vi "Lab_2.vi"() -> ()   [LabVIEW 2021]
panel:
  out "C":dbl[][](array[numeric])
  out "B":dbl[][](array[numeric])
  out "A":dbl[][](array[numeric])
  out "Mo":dbl[][](array[numeric])
  out "Con":dbl[][](array[numeric])
  out "MC":dbl[][](array[numeric])
  in  "b4":dbl
  in  "b3":dbl
  in  "b2":dbl
  in  "b1":dbl
  in  "a4":dbl
  in  "a3":dbl
  in  "a2":dbl
  in  "a1":dbl
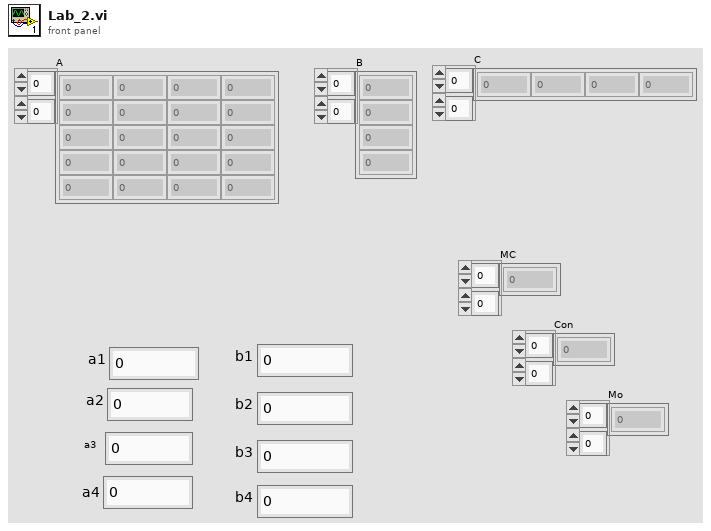
[diagram p1: front panel]
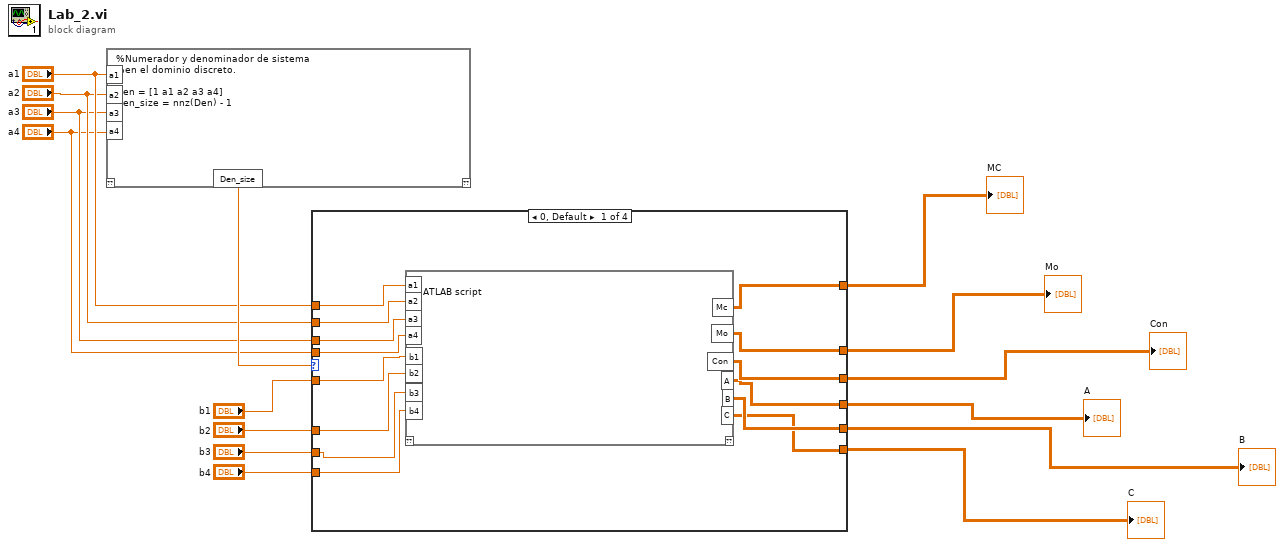
[diagram p0: block diagram]
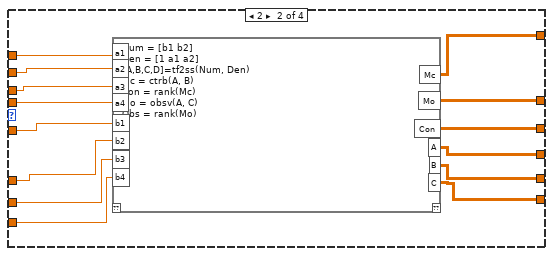
[diagram p2: hidden frame]
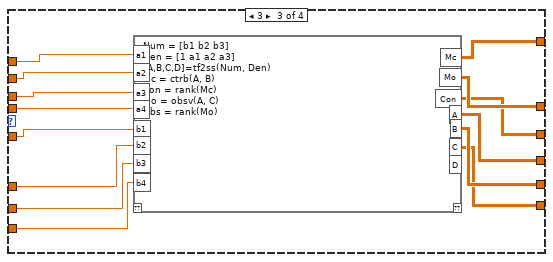
[diagram p3: hidden frame]
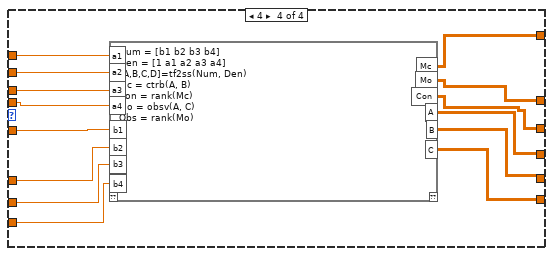
[diagram p4: hidden frame]
diagram:
  n1 = script code="%Numerador y denominador de sistema\n%en el dominio discreto.\n\nDen = [1 a1 a2 a3 a4]\nDen_size = nnz(Den) - 1" ("Script Node")("a1"="a1", "a2"="a2", "a3"="a3", "a4"="a4") -> ("Den_size"=w15:dbl)  [unwired: 1 in, 1 out]
  n2 = case shown="0, Default" w15 {
    tunnel: "b1" -> [w22 w39 w53 w71]
    tunnel: "b2" -> [w21 w38 w52 w70]
    tunnel: "b3" -> [w20 w37 w51 w69]
    tunnel: "b4" -> [w19 w36 w50 w68]
    tunnel: "a1" -> [w26 w43 w57 w67]
    tunnel: "a2" -> [w25 w42 w56 w66]
    tunnel: "a3" -> [w24 w41 w55 w65]
    tunnel: "a4" -> [w23 w40 w54 w64]
    tunnel: [w29 w35 w46 w60] -> w6
    tunnel: [w28 w34 w45 w59] -> w4
    tunnel: [w27 w33 w44 w58] -> w5
    tunnel: [w18 w32 w49 w61] -> w3
    tunnel: [w17 w31 w48 w62] -> w2
    tunnel: [w16 w30 w47 w63] -> w1
    frame 0, Default {
      n3 = script code="MATLAB script"("b1"=w22, "b2"=w21, "b3"=w20, "b4"=w19, "a1"=w26, "a2"=w25, "a3"=w24, "a4"=w23) -> ("Mc"=w29:dbl[][], "Mo"=w28:dbl[][], "Con"=w27:dbl[][], "A"=w18:dbl[][], "B"=w17:dbl[][], "C"=w16:dbl[][])  [unwired: 1 in, 1 out]
    }
    frame 2 {
      n4 = script code="Num = [b1 b2]\nDen = [1 a1 a2]\n[A,B,C,D]=tf2ss(Num, Den)\nMc = ctrb(A, B)\nCon = rank(Mc)\nMo = obsv(A, C)\nObs = rank(Mo)"("b1"=w39, "b2"=w38, "b3"=w37, "b4"=w36, "a1"=w43, "a2"=w42, "a3"=w41, "a4"=w40) -> ("Mc"=w35:dbl[][], "Mo"=w34:dbl[][], "Con"=w33:dbl[][], "A"=w32:dbl[][], "B"=w31:dbl[][], "C"=w30:dbl[][])  [unwired: 1 in, 1 out]
    }
    frame 3 {
      n5 = script code="Num = [b1 b2 b3]\nDen = [1 a1 a2 a3]\n[A,B,C,D]=tf2ss(Num, Den)\nMc = ctrb(A, B)\nCon = rank(Mc)\nMo = obsv(A, C)\nObs = rank(Mo)"("b1"=w53, "b2"=w52, "b3"=w51, "b4"=w50, "a1"=w57, "a2"=w56, "a3"=w55, "a4"=w54) -> ("Mc"=w46:dbl[][], "Mo"=w45:dbl[][], "Con"=w44:dbl[][], "A"=w49:dbl[][], "B"=w48:dbl[][], "C"=w47:dbl[][])  [unwired: 1 in, 2 out]
    }
    frame 4 {
      n6 = script code="Num = [b1 b2 b3 b4]\nDen = [1 a1 a2 a3 a4]\n[A,B,C,D]=tf2ss(Num, Den)\nMc = ctrb(A, B)\nCon = rank(Mc)\nMo = obsv(A, C)\nObs = rank(Mo)"("b1"=w71, "b2"=w70, "b3"=w69, "b4"=w68, "a1"=w67, "a2"=w66, "a3"=w65, "a4"=w64) -> ("Mc"=w60:dbl[][], "Mo"=w59:dbl[][], "Con"=w58:dbl[][], "A"=w61:dbl[][], "B"=w62:dbl[][], "C"=w63:dbl[][])  [unwired: 1 in, 1 out]
    }
  }
  "MC" <- w6
  "Con" <- w5
  "Mo" <- w4
  "A" <- w3
  "B" <- w2
  "C" <- w1
